vi "Point is in Rectangle.vi"(1 "Bounds":T1={"Left"=33, "Top"=22, "Right"=80, "Bottom"=41}, 2 "Point":cluster{"H":T2, "V":T2}) -> (0 "In Bounds?":bool)   [LabVIEW 2012]
uses:
  <vilib>/XNodeSupport/XNodeInt.ctl
  <vilib>/XNodeSupport/XNodeRect32.ctl
  <vilib>/XNodeSupport/NI_XNodeSupport.lvlib
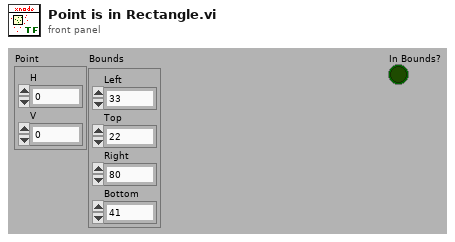
[diagram p1: front panel]
types:
  T1 = typedef "NI_XNodeSupport.lvlib/XNodeRect32.ctl" = cluster{"Left":T2, "Top":T2, "Right":T2, "Bottom":T2}
  T2 = typedef "NI_XNodeSupport.lvlib/XNodeInt.ctl" = i32
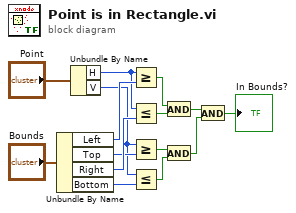
[diagram p0: block diagram]
diagram:
  n1 = Unbundle By Name("Bounds") -> ("Left"=w13:T2, "Top"=w10:T2, "Right"=w11:T2, "Bottom"=w8:T2)
  n2 = Unbundle By Name("Point") -> ("H"=w12:T2, "V"=w9:T2)
  n3 = Greater Or Equal?(x=w12, y=w13) -> (x >= y?=w7:bool)
  n4 = Less Or Equal?(x=w12, y=w11) -> (x <= y?=w6:bool)
  n5 = Greater Or Equal?(x=w9, y=w10) -> (x >= y?=w5:bool)
  n6 = Less Or Equal?(x=w9, y=w8) -> (x <= y?=w4:bool)
  n7 = And(x=w7, y=w6) -> (x .and. y?=w3:bool)
  n8 = And(x=w5, y=w4) -> (x .and. y?=w2:bool)
  n9 = And(x=w3, y=w2) -> (x .and. y?=→"In Bounds?":bool)
